vi "isUniversal.vi"(11 "TopicFilter in":refnum<class "_TopicFilter.lvclass">) -> (2 "universal":bool, 3 "TopicFilter out":refnum<class "_TopicFilter.lvclass">)   [LabVIEW 2013, in "MQTT Server.lvlib" / "_TopicFilter.lvclass"]
uses:
  _TopicFilter.lvclass
  _TopicFilter.lvclass/_TopicFilter.ctl
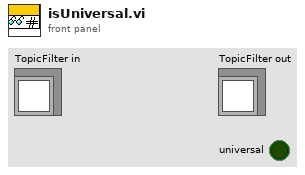
[diagram p1: front panel]
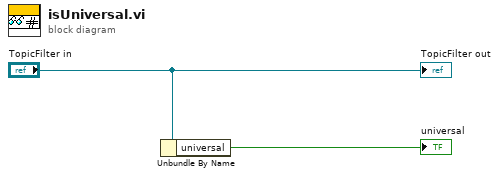
[diagram p0: block diagram]
diagram:
  n1 = Unbundle By Name("TopicFilter in") -> ("universal"=→"universal":bool)
  "TopicFilter out" <- "TopicFilter in"
